vi "ADXL345.vi"() -> ()   [LabVIEW 2019]
uses:
  <vilib>/MakerHub/LINX/Public/Sensors/Accelerometer/MPU60X0/DeviceAddresses.ctl
  <vilib>/MakerHub/LINX/Public/Utilities/Open Serial.vi
  <vilib>/picture/3D Picture Control/Object/Create Object (drawable).vi
  <vilib>/MakerHub/LINX/LMH-LINX.lvlib
  <vilib>/MakerHub/LINX/Public/Sensors/Accelerometer/MPU60X0/MPU60X0.lvlib
  <vilib>/picture/3D Picture Control/NI_3D Picture Control.lvlib
panel:
  in  "Angle":sgl=30.0
  out "3D Picture 2":refnum<vi>(3d-picture)
  out "Acceleration Data (g)":T1
  in  "stop":bool
  in  "Serial Port":refnum<visa-resource-name>="N/A"
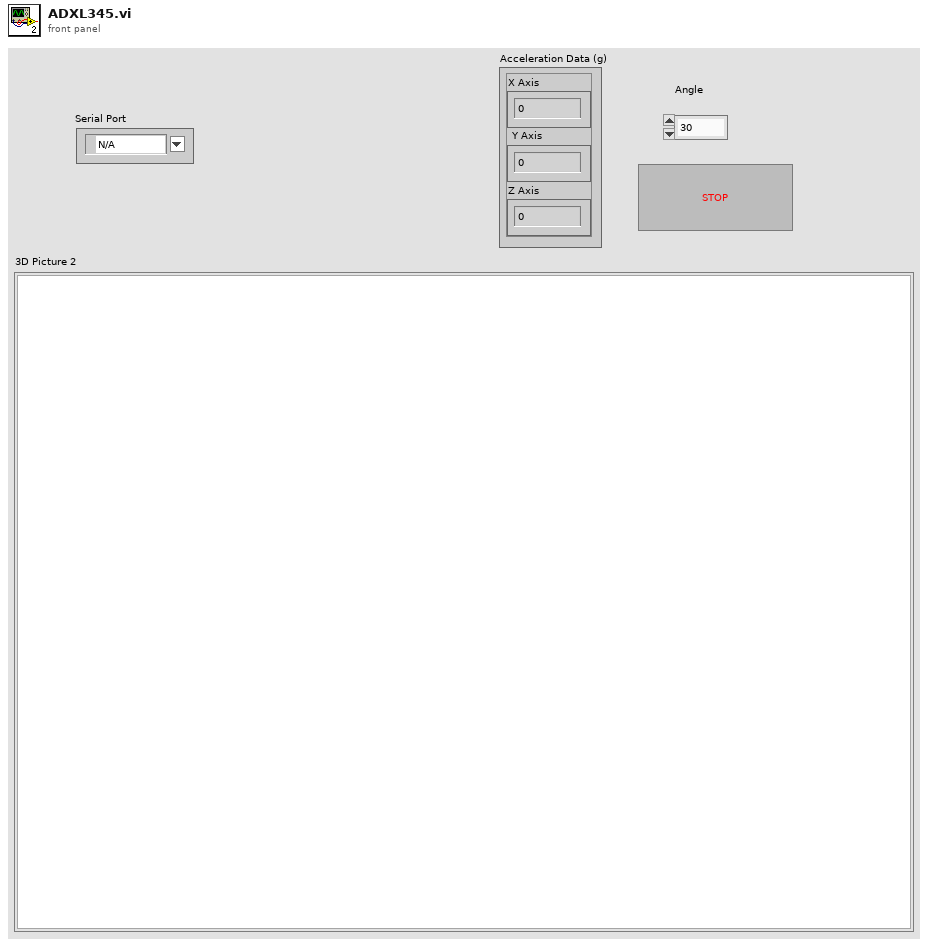
[diagram p1: front panel]
types:
  T1 = cluster{"X Axis":i16, "Y Axis":i16, "Z Axis":i16}
  T2 = typedef "LMH-LINX.lvlib/MPU60X0.lvlib/DeviceAddresses.ctl" = enum16{"0x68", "0x69"}
  T3 = typedef "LMH-LINX.lvlib/LINX Ref.ctl" = cluster{"IO":T4, "Interface":T5, "LINX Device Config":T6}
  T4 = typedef "LMH-LINX.lvlib/Platform.ctl" = enum16{"Remote", "Local"}
  T5 = typedef "LMH-LINX.lvlib/Interface.ctl" = enum16{"Serial", "TCP"}
  T6 = typedef "LMH-LINX.lvlib/Device.lvlib/LINX Device Config.ctl" = cluster{"Interface":T5, "COM Port":refnum<visa-resource-name>, "TCP Configuration":T7, "Device Family":u8, "Device ID":u8, "Device Name":string, "TCP Ref":refnum<k5>, "Channels":T8}
  T7 = typedef "LMH-LINX.lvlib/Device.lvlib/TCP Config.ctl" = cluster{"IP Address":string, "Port":u16}
  T8 = typedef "LMH-LINX.lvlib/Channels.ctl" = cluster{"DI":u8[], "DO":u8[], "AI":u8[], "AO":u8[], "PWM":u8[], "QE":u8[], "UART":u8[], "I2C 2":u8[], "SPI":u8[], "CAN":u8[], "Servo":u8[], "AI Ref (V)":dbl, "AI Resolution (Bits)":u8, "AO Ref (V)":dbl, "AO Resolution (Bits)":u8}
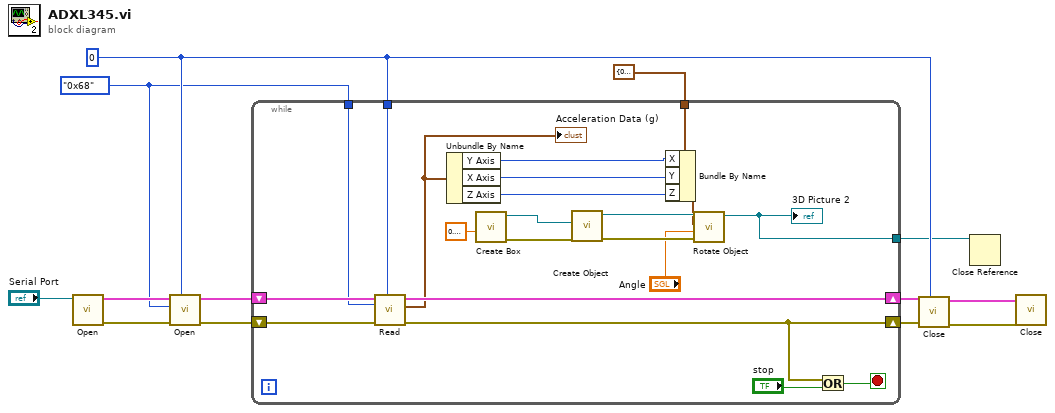
[diagram p0: block diagram]
diagram:
  w4 = u8 0 ("I2C Channel")
  w3 = DeviceAddresses."0x68" ("I2C Slave Address")
  n1 = call-poly <vilib>:"Open.vi"("Serial Port"="Serial Port") -> ("Error Out"=w10:errorcluster, "LINX Resource"=w12:T3)  [unwired: 8 in, 1 out]
  n2 = call <vilib>:"Open.vi"("I2C Channel"=w4, "Error In"=w10, "I2C Slave Address"=w3, "LINX Resource"=w12) -> ("Error Out"=w9:errorcluster, "LINX Resource"=w11:T3)  [unwired: 6 in]
  n3 = while {
    shift-right: [w31] -> w8
    shift-left: w11 -> [w32]
    shift-right: [w29] -> w6
    shift-left: w9 -> [w30]
    tunnel: w3 -> [w28]
    tunnel: w4 -> [w27]
    tunnel: [w21] -> w2
    tunnel: cluster{"X":sgl, "Y":sgl, "Z":sgl} {"X"=0.0, "Y"=0.0, "Z"=0.0} ("Axis") -> [w19]
    stop <- w33 stop-if-true
    n4 = call <vilib>:"Read.vi"("I2C Channel"=w27, "Error In"=w30, "I2C Slave Address"=w28, "LINX Resource"=w32) -> ("Error Out"=w29:errorcluster, "Acceleration Data (g)"=w20:T1, "LINX Resource"=w31:T3)  [unwired: 3 in, 2 out]
    "Acceleration Data (g)" <- w20
    n5 = Unbundle By Name(w20) -> ("Y Axis"=w17:i16, "X Axis"=w16:i16, "Z Axis"=w15:i16)
    n6 = call <vilib>:"Create Box.vi"("Length Z"=sgl 0.2) -> ("error out"=w23:errorcluster, "New Box Refnum"=w22:refnum<vi>)  [unwired: 9 in]
    n7 = call-poly <vilib>:"Create Object.vi"("error in (no error)"=w23, "Geometry"=w22) -> ("error out"=w25:errorcluster, "Scene:New Object"=w26:refnum<vi>)  [unwired: 8 in]
    n8 = Bundle By Name(cluster=w19, "X"=w17, "Y"=w16, "Z"=w15) -> (w18:cluster{"X":sgl, "Y":sgl, "Z":sgl})
    n9 = call <vilib>:"Rotate Object.vi"("error in (no error)"=w25, "Angle"="Angle", "Axis"=w18, "Scene.Object In"=w26) -> ("Scene.Object Out"=w21:refnum<vi>)  [unwired: 6 in, 1 out]
    "3D Picture 2" <- w21
    n10 = Or(x=w29, y="stop") -> (x .or. y?=w33:bool)
  }
  n11 = call <vilib>:"Close.vi"("I2C Channel (0)"=w4, "Error In"=w6, "LINX Resource"=w8) -> ("Error Out"=w5:errorcluster, "LINX Resource"=w7:T3)  [unwired: 7 in]
  n12 = Close Reference(reference=w2) -> ()  [unwired: 1 in, 1 out]
  n13 = call <vilib>:"Close.vi"("Error In"=w5, "LINX Resource"=w7) -> ()  [unwired: 9 in, 1 out]
